vi "Client Send.vi"(8 "error in (no error)":errorcluster, 10 "JSON (UTF-8) String In":string, 11 "Telegram Class in":refnum<class "Telegram Class.lvclass">) -> (0 "error out":errorcluster, 2 "UTF-8 String Out":string, 3 "Telegram Class out":refnum<class "Telegram Class.lvclass">)   [LabVIEW 2015, in "Telegram Library.lvlib" / "Telegram Class.lvclass"]
doc: "Created IvanLis by LabVIEW Portal\nProfile: http://labviewportal.org/memberlist.php?mode=viewprofile&u=987\neMail: IvanLisanov@gMail.com\nTelegram: https://t.me/IvanLis"
uses:
  Telegram Class.lvclass
  Telegram Class.lvclass/Telegram Class.ctl
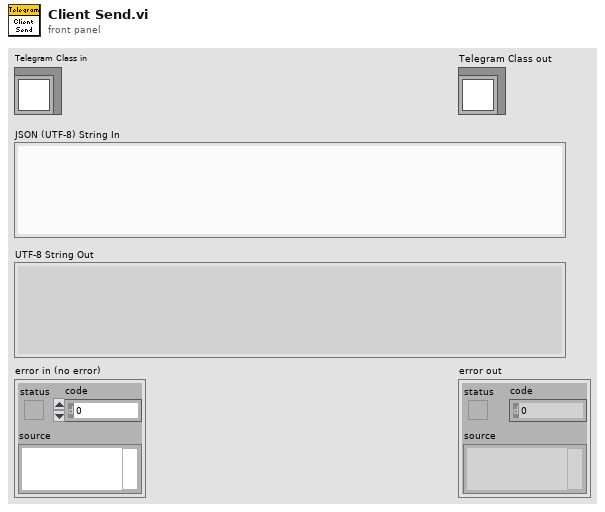
[diagram p1: front panel]
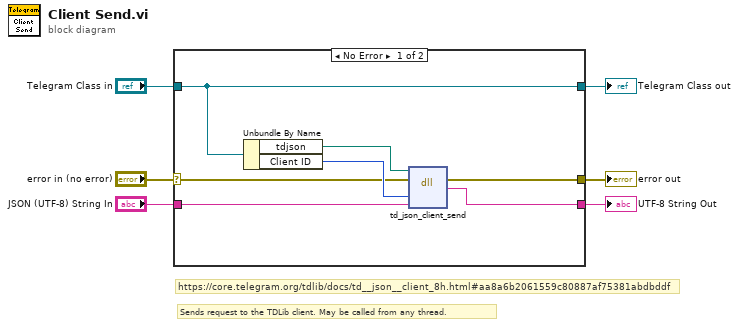
[diagram p0: block diagram]
diagram:
  # "Sends request to the TDLib client. May be called from any thread."
  # "https://core.telegram.org/tdlib/docs/td__json__client_8h.html#aa8a6b2061559c80887af75381abdbddf"
  n1 = case shown="No Error" "error in (no error)" {
    selector: "error in (no error)" -> [w8 w15]
    tunnel: [w10 w15] -> w5
    tunnel: [w13 w14] -> w3
    tunnel: "Telegram Class in" -> [w13 w14]
    tunnel: "JSON (UTF-8) String In" -> [w7 _]
    tunnel: [w9 _] -> w1
    frame No Error {
      n2 = Unbundle By Name(w13) -> ("tdjson"=w12:path, "Client ID"=w11:i32)
      n3 = dll-call lib="C:/Users/Ivan/Desktop/Telegram/Project/DLL/tdjson-x32.dll" fn="td_json_client_send"(path in=w12, error in=w8, "Client ID"=w11, "String"=w7) -> (error out=w10:errorcluster, "String"=w9:string)  [unwired: 3 in, 1 out]
    }
    frame Error {
    }
  }
  "error out" <- w5
  "Telegram Class out" <- w3
  "UTF-8 String Out" <- w1
